vi "LogFileOpenRef.vi"(6 "Pfad":path=path "T:/Projekt_B2G_FABES/B2G/Messprotokolle_B2G1", 7 "file":bool, 8 "error in (no error)":errorcluster, 9 "file reference":refnum<file>, 10 "Output - Cluster":refnum<vi>, 11 "Cluster in":refnum<vi>) -> (0 "error out":errorcluster, 3 "Byte Stream File out":refnum<file>)   [LabVIEW 2011]
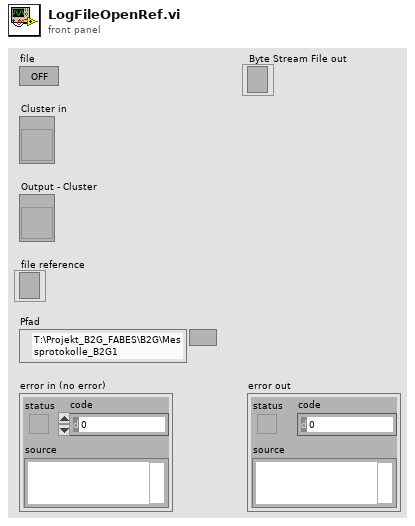
[diagram p1: front panel]
types:
  T1 = enum16{"open", "replace", "create", "open or create", "replace or create", "replace or create with confirmation"}
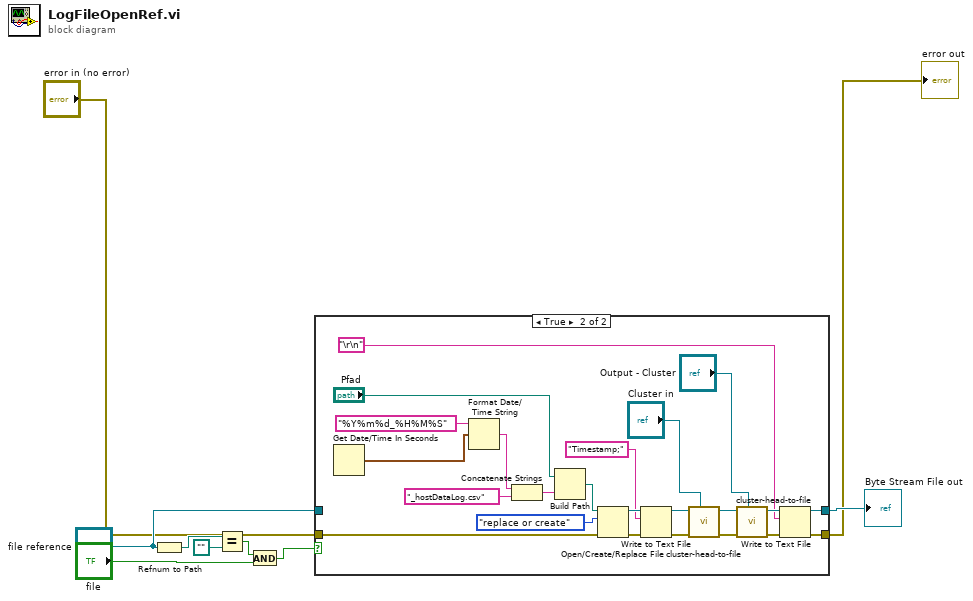
[diagram p0: block diagram]
diagram:
  n1 = Refnum to Path(1:"file reference") -> (0:w2:path)
  n2 = Equal?(x=w2, y=path "") -> (x = y?=w4:bool)
  n3 = And(x=w4, y="file") -> (x .and. y?=w7:bool)
  n4 = case shown="True" w7 {
    tunnel: [w10 w20] -> w9
    tunnel: [w11 w19] -> w8
    tunnel: "error in (no error)" -> [w11 w12]
    tunnel: "file reference" -> [w10 _]
    frame False {
    }
    frame True {
      n5 = Get Date/Time In Seconds() -> (seconds since 1Jan1904=w32:timestamp)
      n6 = Format Date/Time String(time format string (%c)="%Y%m%d_%H%M%S", seconds (now)=w32) -> (date/time string=w31:string)  [unwired: 1 in]
      n7 = Concatenate Strings(w31, "_hostDataLog.csv" ("name or relative path")) -> (w28:string)
      n8 = Build Path(base path="Pfad", name or relative path=w28) -> (appended path=w27:path)
      n9 = Open/Create/Replace File(file path (use dialog)=w27, error in=w12, operation (0:open)=T1."replace or create") -> (refnum out=w17:refnum<file>, error out=w16:errorcluster)  [unwired: 3 in, 1 out]
      n10 = Write to Text File(file (use dialog)=w17, text="Timestamp;", error in=w16) -> (refnum out=w14:refnum<file>, error out=w15:errorcluster)  [unwired: 1 in, 1 out]
      n11 = call "cluster-head-to-file.vi"("refnum in"=w14, "error in"=w15, "cluster ref"="Cluster in") -> ("refnum out"=w25:refnum<file>, "error out"=w24:errorcluster)  [unwired: 6 in]
      n12 = call "cluster-head-to-file.vi"("refnum in"=w25, "error in"=w24, "cluster ref"="Output - Cluster") -> ("refnum out"=w22:refnum<file>, "error out"=w21:errorcluster)  [unwired: 6 in]
      n13 = Write to Text File(file (use dialog)=w22, text="\r\n", error in=w21) -> (refnum out=w20:refnum<file>, error out=w19:errorcluster)  [unwired: 1 in, 1 out]
    }
  }
  "Byte Stream File out" <- w9
  "error out" <- w8
